vi "CharToAscii(cast).vi"(1 "Char":string) -> (0 "ASCII":u8 format="DEC:%2d\nHEX:%2x")   [LabVIEW 2012]
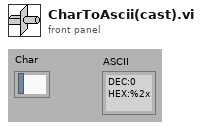
[diagram p1: front panel]
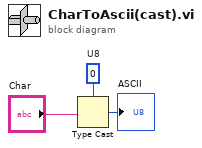
[diagram p0: block diagram]
diagram:
  w2 = u8 0  # U8
  n1 = Type Cast(type=w2, x="Char") -> (*(type *) &x=→"ASCII":u8)
